vi "Drag Over (inline).vi"(8 "error in (no error)":errorcluster, 9 "Coords":T1, 10 "BetterDropOp":refnum<class "BetterDropOp.lvclass">, 11 "BetterHandle in":refnum<class "BetterHandle.lvclass">) -> (0 "error out":errorcluster, 2 "Drag Accepted?":bool, 3 "BetterHandle out":refnum<class "BetterHandle.lvclass">)   [LabVIEW 2020, in "BetterDragAndDrop.lvlib" / "BetterHandle.lvclass"]
uses:
  BetterHandle.lvclass
  BetterDropOp/BetterDropOp.lvclass
  <vilib>/Utility/miscctls.llb/LVPoint32TypeDef.ctl
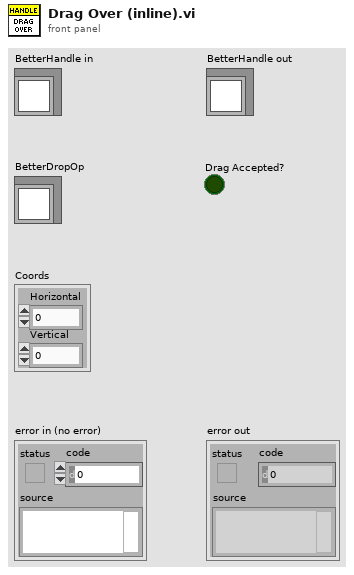
[diagram p1: front panel]
types:
  T1 = typedef "LVPoint32TypeDef.ctl" = cluster{"Horizontal":i32, "Vertical":i32}
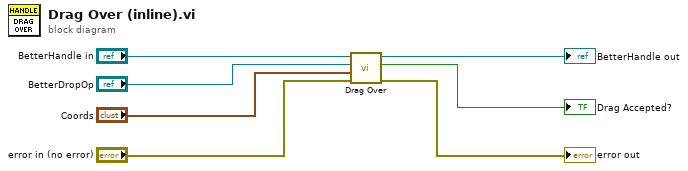
[diagram p0: block diagram]
diagram:
  n1 = call "Drag Over.vi"("error in (no error)"="error in (no error)", "Coords"="Coords", "BetterDropOp"="BetterDropOp", "BetterHandle in"="BetterHandle in") -> ("error out"=→"error out":errorcluster, "Drag Accepted?"=→"Drag Accepted?":bool, "BetterHandle out"=→"BetterHandle out":refnum<class "BetterHandle.lvclass">)  [unwired: 5 in]
